vi "CreateLicTool.vi"() -> ()   [LabVIEW 2013]
panel:
  in  "退出按钮":bool
  in  "确定按钮":bool
  out "大小 4":i32
  out "大小 3":i32
  out "大小 2":i32
  out "大小":i32
  in  "LicCode":string
  in  "簇":T1
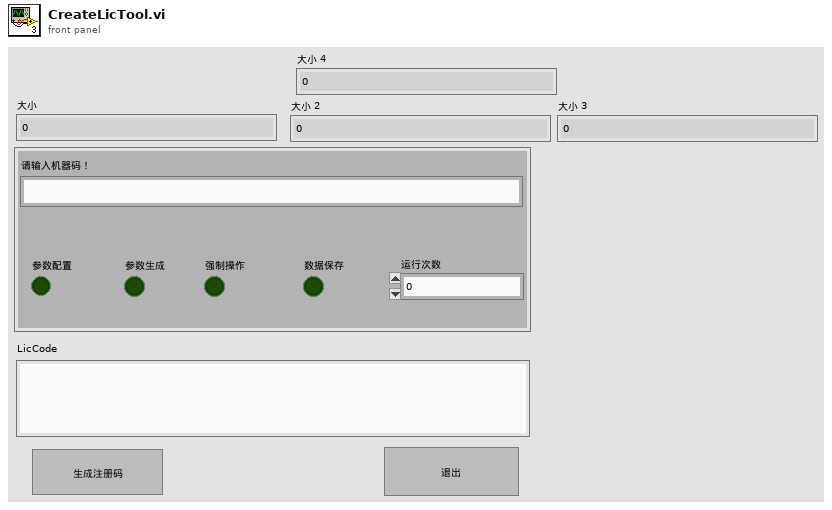
[diagram p1: front panel]
types:
  T1 = cluster{"请输入机器码！":string, "LicCode":string, "运行次数":dbl, "StartTime":string, "EndTime":string, "参数配置":bool, "参数生成":bool, "强制操作":bool, "数据保存":bool}
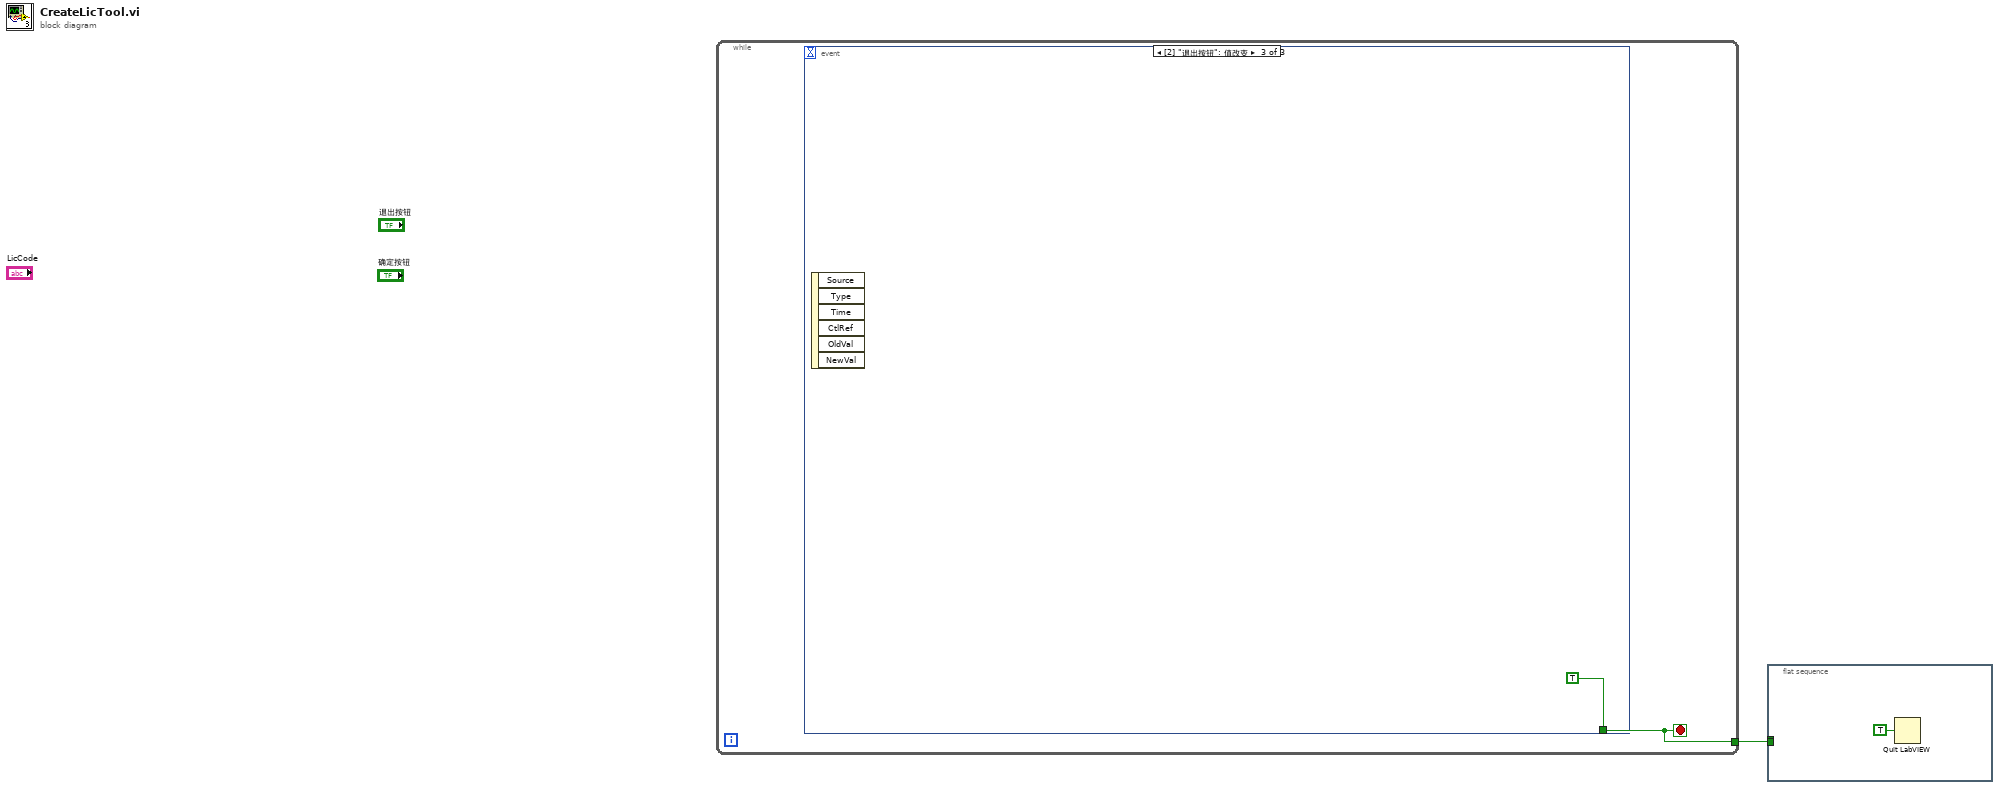
[diagram p0: block diagram]
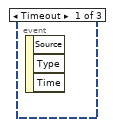
[diagram p2: hidden frame]
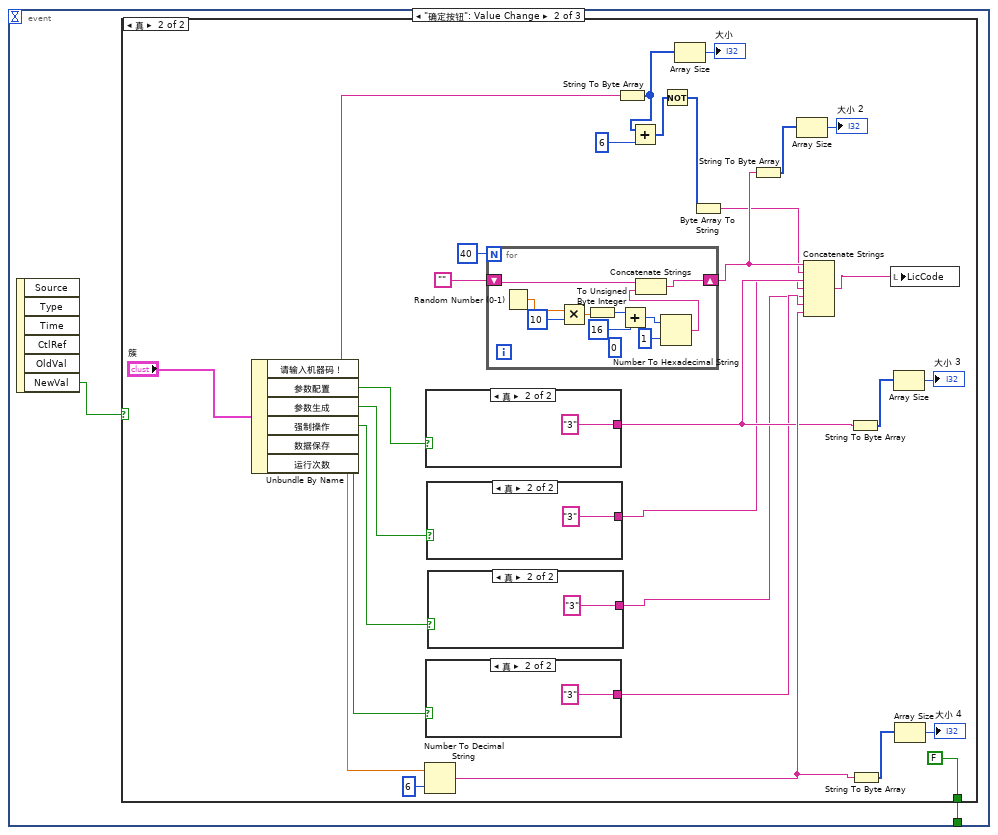
[diagram p3: hidden frame]
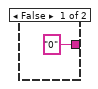
[diagram p5: hidden frame]
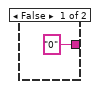
[diagram p6: hidden frame]
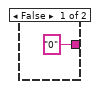
[diagram p7: hidden frame]
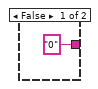
[diagram p8: hidden frame]
diagram:
  n1 = while {
    tunnel: [w2] -> w1
    stop <- w2 stop-if-true
    n2 = event shown="[2] \"退出按钮\": 值改变" {
      selector: _ -> [_ _ _]
      dyn-events: _ -> [_ _ _]
      timeout: _ -> [_ _ _]
      tunnel: [_ w3 TRUE] -> w2
      event Timeout {
        n3 = event-data() -> ()  [unwired: 1 in, 3 out]
      }
      event "确定按钮": Value Change {
        n4 = event-data() -> ("NewVal"=w4:bool)  [unwired: 1 in, 5 out]
        n5 = case shown="真" w4 {
          tunnel: [_ FALSE] -> w3
          frame False {
          }
          frame True {
            n6 = Unbundle By Name("簇") -> ("请输入机器码！"=w11:string, "参数配置"=w12:bool, "参数生成"=w13:bool, "强制操作"=w14:bool, "数据保存"=w15:bool, "运行次数"=w19:dbl)
            n7 = Number To Decimal String(number=w19, width (-)=i16 6 ("宽度(-)")) -> (decimal integer string=w33:string)
            n8 = case shown="真" w12 {
              tunnel: ["0" ("字符串") "3" ("字符串")] -> w30
              frame False {
              }
              frame True {
              }
            }
            n9 = case shown="真" w15 {
              tunnel: ["0" ("字符串") "3" ("字符串")] -> w18
              frame False {
              }
              frame True {
              }
            }
            n10 = case shown="真" w13 {
              tunnel: ["0" ("字符串") "3" ("字符串")] -> w16
              frame False {
              }
              frame True {
              }
            }
            n11 = case shown="真" w14 {
              tunnel: ["0" ("字符串") "3" ("字符串")] -> w17
              frame False {
              }
              frame True {
              }
            }
            n12 = for {
              N: 40 -> [_]
              shift-right: [w44] -> w25
              shift-left: "" -> [w45]
              (unwired) 0 ("数字")
              n13 = Random Number (0-1)() -> (number: 0 to 1=w51:dbl)
              n14 = Multiply(x=w51, y=u8 10) -> (x*y=w49:dbl)
              n15 = To Unsigned Byte Integer(number=w49) -> (unsigned 8bit integer=w47:u8)
              n16 = Add(x=w47, y=u8 16) -> (x+y=w42:u8)
              n17 = Number To Hexadecimal String(1:i16 1 ("宽度(-)"), 2:w42) -> (0:w43:string)
              n18 = Concatenate Strings(w45, w43) -> (w44:string)
            }
            n19 = String To Byte Array(string=w11) -> (unsigned byte array=w23:u8[])
            n20 = Add(x=w23, y=u8 6) -> (x+y=w9:u8[])
            n21 = Not(x=w9) -> ()  [unwired: 1 out]
            n22 = Array Size(array=w23) -> (size(s)=→"大小":i32)
            n23 = Byte Array To String(unsigned byte array=w9) -> (string=w22:string)
            n24 = String To Byte Array(string=w25) -> (unsigned byte array=w27:u8[])
            n25 = Array Size(array=w27) -> (size(s)=→"大小 2":i32)
            n26 = Concatenate Strings(w25, w22, w30, w16, w17, w18, w33) -> (w21:string)
            n27 = String To Byte Array(string=w30) -> (unsigned byte array=w28:u8[])
            n28 = String To Byte Array(string=w33) -> (unsigned byte array=w32:u8[])
            n29 = local write "LicCode"(w21) -> ()
            n30 = Array Size(array=w28) -> (size(s)=→"大小 3":i32)
            n31 = Array Size(array=w32) -> (size(s)=→"大小 4":i32)
          }
        }
      }
      event "退出按钮": Value Change {
        n32 = event-data() -> ()  [unwired: 1 in, 6 out]
      }
    }
  }
  n33 = flat-sequence {
    tunnel: [w54] -> _
    tunnel: w1 -> [w54]
    frame #0 {
      n34 = Quit LabVIEW(quit? (T)=TRUE ("退出？(T)")) -> ()
    }
  }
